vi "CreatePrivateEvents.vi"(8 "error in (no error)":errorcluster, 11 "Maui 2.0":refnum<class "Maui 2.0.lvclass">) -> (0 "error out":errorcluster, 3 "Maui 2.0 out":refnum<class "Maui 2.0.lvclass">)   [LabVIEW 2019, in "Maui 2.0.lvclass"]
doc: "---------------------------------------------------------------\nJKI State Machine Objects™\nhttp://jki.net/state-machine-objects/\nCopyright (C) 2005-2015, JKI <info@jki.net>\nALL RIGHTS RESERVEDJKI State Machine Objects (SMO) 1.0.0.4\nJKI - JKI\nCopyright (c) 2015, JKI"
uses:
  Maui 2.0.lvclass
  <vilib>/JKI/JKI SMO/SMO/SMO.lvclass
  Typedefs/PrivateEvents--Maui 2.0.Set Subpanels.ctl
  Typedefs/PrivateEvents--Maui 2.0.Get Subpanels.ctl
  Typedefs/PrivateEvents--Maui 2.0.Set Panels.ctl
panel:
  # "For instructions on how to use the JKI State Machine Objects, examples and video tutorials, visit:\nhttp://jki.net/state-machine-objects/\n\nJKI State Machine Objects™\nhttp://jki.net/state-machine-objects/\nCopyright (C) 2005-2015, JKI <info@jki.net>\nALL RIGHTS RESERVED"
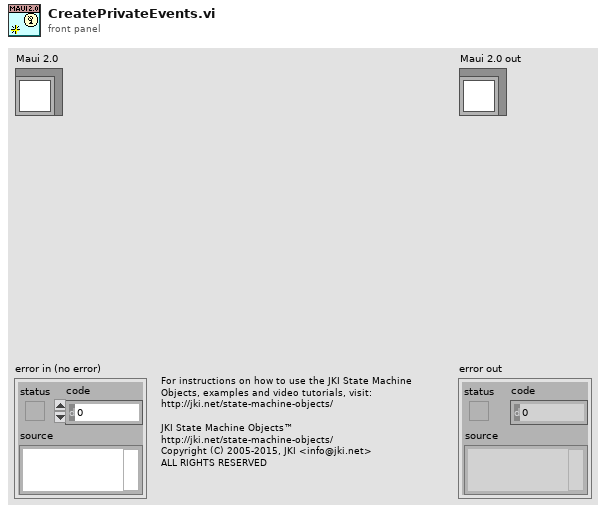
[diagram p1: front panel]
types:
  T1 = typedef "Maui 2.0.lvclass/PrivateEvents--Maui 2.0.Set Panels.ctl" = cluster{"Control":refnum<vi>, "SubPnl":refnum<vi>}[]
  T2 = typedef "Maui 2.0.lvclass/PrivateEvents--Maui 2.0.Get Subpanels.ctl" = refnum<notifier>
  T3 = typedef "Maui 2.0.lvclass/PrivateEvents--Maui 2.0.Set Subpanels.ctl" = cluster{"Subpanels":refnum<class "SMO.lvclass">[], "Append":bool}
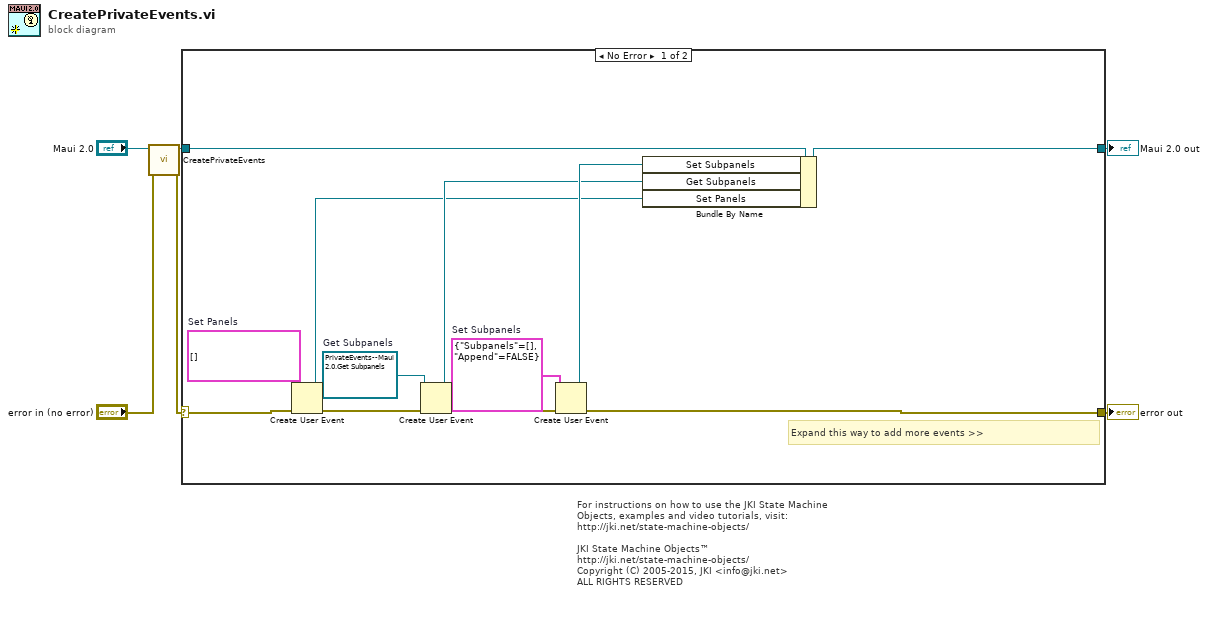
[diagram p0: block diagram]
diagram:
  # "For instructions on how to use the JKI State Machine Objects, examples and video tutorials, visit:\nhttp://jki.net/state-machine-objects/\n\nJKI State Machine Objects™\nhttp://jki.net/state-machine-objects/\nCopyright (C) 2005-2015, JKI <info@jki.net>\nALL RIGHTS RESERVED"
  n1 = call-parent "CreatePrivateEvents.vi"("error in (no error)"="error in (no error)", "SMO"="Maui 2.0") -> ("error out"=w1:errorcluster, "SMO out"=w3:refnum<class "Maui 2.0.lvclass">)  [unwired: 8 in]
  n2 = case shown="No Error" w1 {
    selector: w1 -> [w17 w20]
    tunnel: [w15 w20] -> w5
    tunnel: [w16 w19] -> w6
    tunnel: w3 -> [w18 w19]
    frame No Error {
      w8 = T1 []  # Set Panels
      w11 = T2 refnum  # Get Subpanels
      w14 = T3 {"Subpanels"=[], "Append"=FALSE}  # Set Subpanels
      # "Expand this way to add more events >>"
      n3 = Create User Event(user event datatype=w8, error in=w17) -> (user event=w7:refnum<user-event>, error out=w9:errorcluster)
      n4 = Create User Event(user event datatype=w11, error in=w9) -> (user event=w10:refnum<user-event>, error out=w12:errorcluster)
      n5 = Create User Event(user event datatype=w14, error in=w12) -> (user event=w13:refnum<user-event>, error out=w15:errorcluster)
      n6 = Bundle By Name(cluster=w18, "Set Subpanels"=w13, "Get Subpanels"=w10, "Set Panels"=w7) -> (w16:refnum<class "Maui 2.0.lvclass">)
    }
    frame Error {
    }
  }
  "error out" <- w5
  "Maui 2.0 out" <- w6
